vi "writeFactorPass.vi"(6 "Pass?":bool, 8 "error in (no error)":errorcluster, 9 "FactorPass in":cluster{"id":dbl[], "value":dbl[]}, 10 "Game in":refnum<class "Game.lvclass">, 11 "Utilities in":refnum<class "Utilities.lvclass">) -> (0 "error out":errorcluster, 1 "Debug":dbl[][](array[numeric]), 2 "FactorPass out":cluster{"id":dbl[], "value":dbl[]}, 3 "Utilities out":refnum<class "Utilities.lvclass">, 4 "FactorPass":dbl[](array[numeric]))   [LabVIEW 2021, in "Utilities.lvclass"]
uses:
  Utilities.lvclass
  Game_class/Game.lvclass
  Enemy_class/Enemy.lvclass
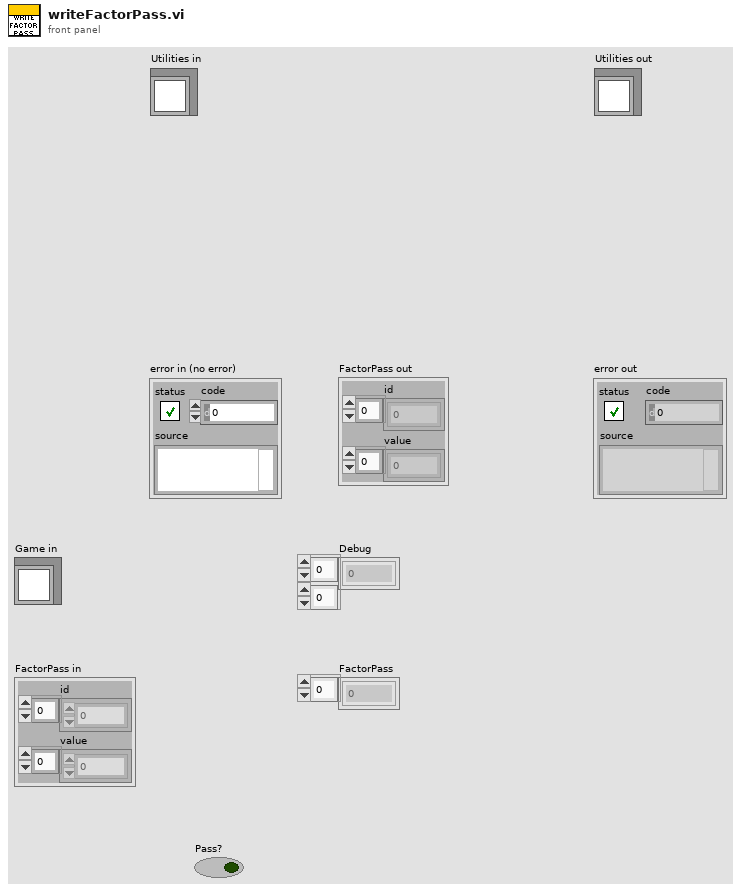
[diagram p1: front panel]
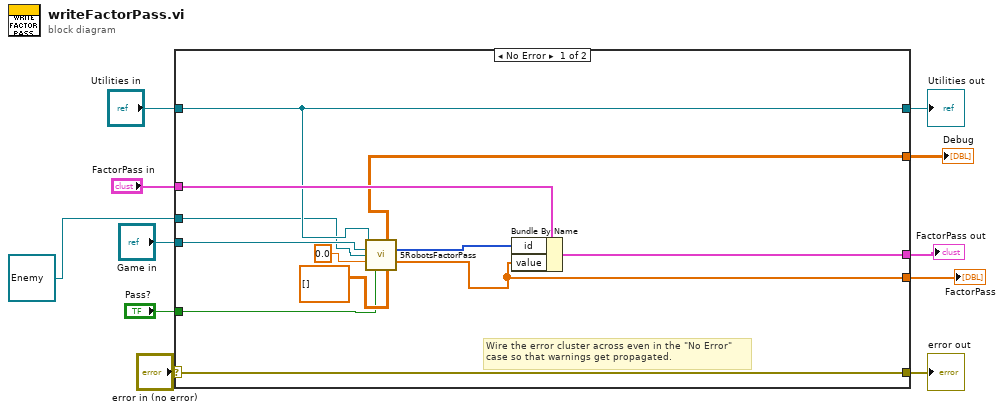
[diagram p0: block diagram]
diagram:
  n1 = case shown="No Error" "error in (no error)" {
    selector: "error in (no error)" -> [w23 w25]
    tunnel: [w23 w25] -> w10
    tunnel: [w20 w24] -> w8
    tunnel: "Utilities in" -> [w20 w24]
    tunnel: [w19 _] -> w7
    tunnel: [w22 _] -> w6
    tunnel: [w17 _] -> w5
    tunnel: "Game in" -> [w13 _]
    tunnel: "FactorPass in" -> [w21 _]
    tunnel: "Pass?" -> [w14 _]
    tunnel: refnum<class "Enemy.lvclass"> refnum ("reference") -> [w12 _]
    frame No Error {
      # "Wire the error cluster across even in the \"No Error\"\ncase so that warnings get propagated."
      n2 = call-dynamic "5RobotsFactorPass.vi"("Utilities in"=w20, "Game in"=w13, "reference"=w12, "Root"=0.0, "Pass?"=w14, "dest_kick"=dbl[][] []) -> ("Debug"=w19:dbl[][], "Id"=w18:i32[], "FactorPass"=w17:dbl[])  [unwired: 5 in, 2 out]
      n3 = Bundle By Name(cluster=w21, "id"=w18, "value"=w17) -> (w22:cluster{"id":dbl[], "value":dbl[]})
    }
    frame Error {
    }
  }
  "error out" <- w10
  "Utilities out" <- w8
  "Debug" <- w7
  "FactorPass out" <- w6
  "FactorPass" <- w5
